vi "Secondary Xbox.vi"(10 "Secondary":T3, 11 "Dash Data In":T2={"Joy Stick"={"Primary"={"Buttons"={"A"=FALSE, "B"=FALSE, "X"=FALSE, "Y"=FALSE, "Left Bumper"=FALSE, "Right Bumper"=FALSE, "Back"=FALSE, "Start"=FALSE, "Left Thumbstick"=FALSE, "Right Thumbstick"=FALSE}, "Axes"={"Left Stick X "=0.0, "Left Stick Y"=0.0, "Triggers"=-0.0, "Right Stick X"=0.0, "Right Stick Y"=0.0, "D-Pad X"=0.0}}, "Secondary"={"Buttons"={"A"=FALSE, "B"=FALSE, "X"=FALSE, "Y"=FALSE, "Left Bumper"=FALSE, "Right Bumper"=FALSE, "Back"=FALSE, "Start"=FALSE, "Left Thumbstick"=FALSE, "Right Thumbstick"=FALSE}, "Axes"={"Left Stick X "=0.0, "Left Stick Y"=0.0, "Triggers"=0.0, "Right Stick X"=0.0, "Right Stick Y"=0.0, "D-Pad X"=0.0}}}, "Shooter"={"RPM Current"=0.0, "RPM Set"=0.0, "In Range?"=FALSE}, "Arm"={"Arm Current"=0.0, "Arm Set"=0.0, "At Position?"=FALSE, "Reset Encoder"=FALSE}, "Drive"={"Right"=0.0, "Left"=0.0}, "Climb State"=enum."Arm Attach", "Change Retical"=FALSE, "Solenoids"={"Robot Angle"=enum."Off", "Shooter Angle"=enum."Off", "Arm Lock"=enum."Off"}, "Shooter Speeds"=[]}) -> (3 "Dash Data Out 2":T2={"Joy Stick"={"Primary"={"Buttons"={"A"=FALSE, "B"=FALSE, "X"=FALSE, "Y"=FALSE, "Left Bumper"=FALSE, "Right Bumper"=FALSE, "Back"=FALSE, "Start"=FALSE, "Left Thumbstick"=FALSE, "Right Thumbstick"=FALSE}, "Axes"={"Left Stick X "=0.0, "Left Stick Y"=0.0, "Triggers"=-0.0, "Right Stick X"=0.0, "Right Stick Y"=0.0, "D-Pad X"=0.0}}, "Secondary"={"Buttons"={"A"=FALSE, "B"=FALSE, "X"=FALSE, "Y"=FALSE, "Left Bumper"=FALSE, "Right Bumper"=FALSE, "Back"=FALSE, "Start"=FALSE, "Left Thumbstick"=FALSE, "Right Thumbstick"=FALSE}, "Axes"={"Left Stick X "=0.0, "Left Stick Y"=0.0, "Triggers"=0.0, "Right Stick X"=0.0, "Right Stick Y"=0.0, "D-Pad X"=0.0}}}, "Shooter"={"RPM Current"=0.0, "RPM Set"=0.0, "In Range?"=FALSE}, "Arm"={"Arm Current"=0.0, "Arm Set"=0.0, "At Position?"=FALSE, "Reset Encoder"=FALSE}, "Drive"={"Right"=0.0, "Left"=0.0}, "Climb State"=enum."Arm Attach", "Change Retical"=FALSE, "Solenoids"={"Robot Angle"=enum."Off", "Shooter Angle"=enum."Off", "Arm Lock"=enum."Off"}, "Shooter Speeds"=[]})   [LabVIEW 2012]
uses:
  <vilib>/Rock Robotics/WPI/Solenoid/WPI_SolenoidValue.ctl
types:
  T1 = typedef "WPI_SolenoidValue.ctl" = enum16{"Off", "On", "Forward", "Reverse"}
  T2 = cluster{"Joy Stick":cluster{"Primary":cluster{"Buttons":cluster{"A":bool, "B":bool, "X":bool, "Y":bool, "Left Bumper":bool, "Right Bumper":bool, "Back":bool, "Start":bool, "Left Thumbstick":bool, "Right Thumbstick":bool}, "Axes":cluster{"Left Stick X ":dbl, "Left Stick Y":dbl, "Triggers":dbl, "Right Stick X":dbl, "Right Stick Y":dbl, "D-Pad X":dbl}}, "Secondary":cluster{"Buttons":cluster{"A":bool, "B":bool, "X":bool, "Y":bool, "Left Bumper":bool, "Right Bumper":bool, "Back":bool, "Start":bool, "Left Thumbstick":bool, "Right Thumbstick":bool}, "Axes":cluster{"Left Stick X ":dbl, "Left Stick Y":dbl, "Triggers":dbl, "Right Stick X":dbl, "Right Stick Y":dbl, "D-Pad X":dbl}}}, "Shooter":cluster{"RPM Current":dbl, "RPM Set":dbl, "In Range?":bool}, "Arm":cluster{"Arm Current":dbl, "Arm Set":dbl, "At Position?":bool, "Reset Encoder":bool}, "Drive":cluster{"Right":dbl, "Left":dbl}, "Climb State":enum16{"Arm Wait", "Arm Up", "Arm Down", "Arm Attach"}, "Change Retical":bool, "Solenoids":cluster{"Robot Angle":T1, "Shooter Angle":T1, "Arm Lock":T1}, "Shooter Speeds":dbl[]}
  T3 = cluster{"Buttons":cluster{"A":bool, "B":bool, "X":bool, "Y":bool, "Left Bumper":bool, "Right Bumper":bool, "Back":bool, "Start":bool, "Left Thumbstick":bool, "Right Thumbstick":bool}, "Axes":cluster{"Left Stick X ":dbl, "Left Stick Y":dbl, "Triggers":dbl, "Right Stick X":dbl, "Right Stick Y":dbl, "D-Pad X":dbl}}
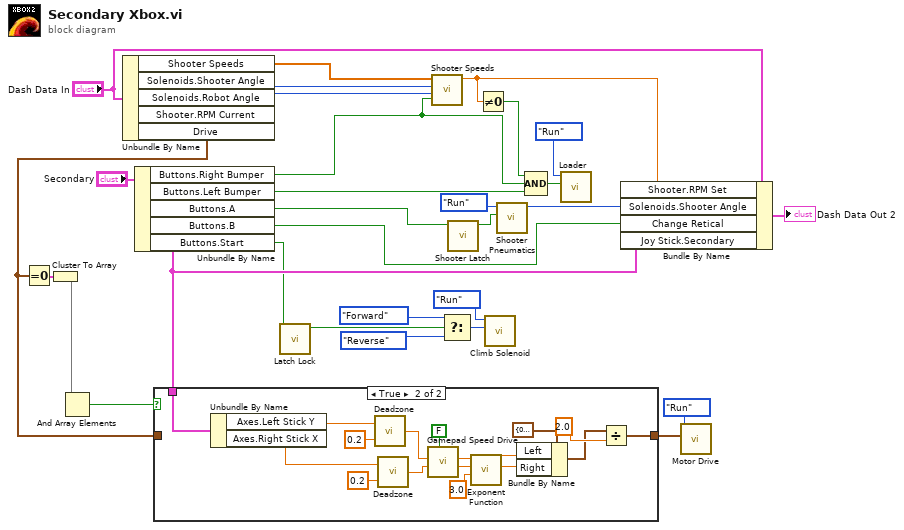
[diagram p0: block diagram]
diagram:
  n1 = Unbundle By Name("Dash Data In") -> ("Shooter Speeds"=w23:dbl[], "Solenoids.Shooter Angle"=w20:T1, "Solenoids.Robot Angle"=w22:T1, "Drive"=w14:cluster{"Right":dbl, "Left":dbl})  [unwired: 1 out]
  n2 = Equal To 0?(x=w14) -> (x = 0?=w15:cluster{"Right":bool, "Left":bool})
  n3 = Cluster To Array(cluster=w15) -> (array=w13:bool[])
  n4 = And Array Elements(Boolean array=w13) -> (logical AND=w12:bool)
  n5 = Unbundle By Name("Secondary") -> ("Buttons.Right Bumper"=w11:bool, "Buttons.Left Bumper"=w9:bool, "Buttons.A"=w8:bool, "Buttons.B"=w7:bool, "Buttons.Start"=w1:bool)
  n6 = case shown="True" w12 {
    tunnel: "Secondary" -> [_ w36]
    tunnel: [w30 w32] -> w16
    tunnel: w14 -> [w30 _]
    frame False {
    }
    frame True {
      n7 = Unbundle By Name(w36) -> ("Axes.Left Stick Y"=w35:dbl, "Axes.Right Stick X"=w34:dbl)
      n8 = call "Deadzone.vi"("Deadzone"=0.2, "Input"=w35) -> ("Output"=w43:dbl)
      n9 = call "Deadzone.vi"("Deadzone"=0.2, "Input"=w34) -> ("Output"=w41:dbl)
      n10 = call "Gamepad Speed Drive.vi"("Quick Turn"=FALSE, "Turn"=w41, "Speed"=w43) -> ("Right Output"=w46:dbl, "Left Output"=w47:dbl)  [unwired: 7 in]
      n11 = call "Exponent Function.vi"("Exponent"=3.0, "Left In"=w46, "Right In"=w47) -> ("Right Out"=w38:dbl, "Left Out"=w39:dbl)  [unwired: 7 in]
      n12 = Bundle By Name(cluster=cluster{"Right":dbl, "Left":dbl} {"Right"=0.0, "Left"=0.0} ("Motor"), "Left"=w39, "Right"=w38) -> (w33:cluster{"Right":dbl, "Left":dbl})
      n13 = Divide(x=w33, y=2.0) -> (x/y=w32:cluster{"Right":dbl, "Left":dbl})
    }
  }
  n14 = call "Latch Lock.vi"("Input"=w1) -> ("Latched"=w3:bool)  [unwired: 10 in]
  n15 = call "Shooter Speeds.vi"("Right Bumper"=w11, "Robot Angle"=w22, "Shooter Angle"=w20, "Shooter Speeds"=w23) -> ("f"=w21:dbl)  [unwired: 7 in]
  n16 = Select(t=WPI_SolenoidValue."Forward" ("Value"), s=w3, f=WPI_SolenoidValue."Reverse" ("Value")) -> (s? t:f=w6:T1)
  n17 = call "Shooter Latch.vi"("Input"=w8) -> ("Latched"=w29:bool)  [unwired: 10 in]
  n18 = Not Equal To 0?(x=w21) -> (x != 0?=w10:bool)
  n19 = call "Climb Solenoid.vi"("Value"=w6, "Enum"=enum16{"Start", "Run", "End"}."Run") -> ()  [unwired: 10 in]
  n20 = call "Shooter Pneumatics.vi"("Boolean"=w29, "Enum"=enum16{"Start", "Run", "End"}."Run") -> ("Shooter Angle"=w26:T1)  [unwired: 9 in]
  n21 = Compound Arithmetic op=AND(w10, w11, w9) -> (w19:bool)
  n22 = call "Loader.vi"("Enum"=enum16{"Start", "Run", "End"}."Run", "Run"=w19) -> ()  [unwired: 9 in]
  n23 = Bundle By Name(cluster="Dash Data In", "Shooter.RPM Set"=w21, "Solenoids.Shooter Angle"=w26, "Change Retical"=w7, "Joy Stick.Secondary"="Secondary") -> (→"Dash Data Out 2":T2)
  n24 = call "Motor Drive.vi"("Motor"=w16, "Enum"=enum16{"Start", "Run", "End"}."Run") -> ()  [unwired: 10 in]
